vi "Pre Launch Init.vi"(11 "Popup ViewManager in":refnum<class "Popup ViewManager.lvclass">) -> (0 "error out":errorcluster, 3 "Popup ViewManager out":refnum<class "Popup ViewManager.lvclass">)   [LabVIEW 2019, in "Popup ViewManager.lvlib" / "Popup ViewManager.lvclass"]
doc: "(<B>Filename</B>: Actor Framework.lvlib:Actor.lvclass:Pre Launch Init.vi)\n\nDefines behavior that occurs after the Launch Nested Actor method is invoked but before the actor's Actor Core method begins running.\n\nBy default, this method does nothing. A descendant class may override it to define behavior."
uses:
  <vilib>/gpm_packages/@cs/popup-viewmanager/Source/Popup ViewManager/Popup ViewManager.lvclass
  C:/Program Files/National Instruments/LabVIEW 2019/vi.lib/ActorFramework/Actor/Actor.lvclass
  <vilib>/ActorFramework/Message Enqueuer/Message Priority.ctl
  <vilib>/ActorFramework/Actor/Actor.lvclass/Actor.ctl
  <vilib>/ActorFramework/Message Enqueuer/Message Enqueuer.lvclass/Message Enqueuer.ctl
  <vilib>/gpm_packages/@cs/popup-viewmanager/Source/Popup ViewManager/Popup ViewManager.lvclass/Popup ViewManager.ctl
  <vilib>/ActorFramework/Message Enqueuer/Init from Existing Queue.vi
  <vilib>/ActorFramework/Message Enqueuer/Enqueue.vi
  <vilib>/gpm_packages/@cs/popup-viewmanager/Source/Popup ViewManager Messages/Launch Nested Views Msg/Launch Nested Views Msg.lvclass
  C:/Program Files/National Instruments/LabVIEW 2019/vi.lib/ActorFramework/Message/Message.lvclass
  <vilib>/ActorFramework/Message Priority Queue/Priority Enqueue.vi
  <vilib>/gpm_packages/@cs/mva-dialogbox/source/IDialogBox/IDialogBox/IDialogBox.lvclass
  <vilib>/ActorFramework/Message Enqueuer/Message Enqueuer.lvclass
  <vilib>/ActorFramework/Actor/Actor.lvclass
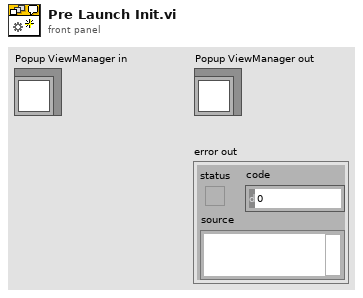
[diagram p1: front panel]
types:
  T1 = typedef "Actor Framework.lvlib/Message Enqueuer.lvclass/Message Priority.ctl" = enum16{"Low", "Normal", "High"}
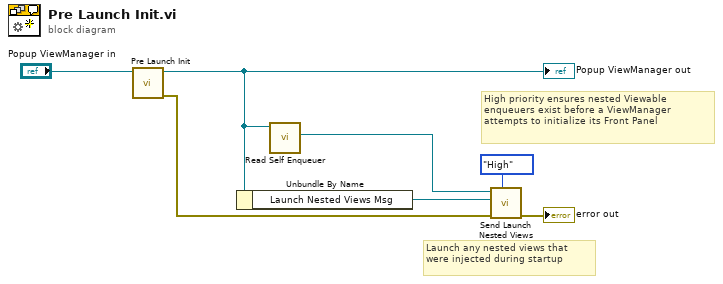
[diagram p0: block diagram]
diagram:
  # "Launch any nested views that\nwere injected during startup"
  # "High priority ensures nested Viewable\nenqueuers exist before a ViewManager\nattempts to initialize its Front Panel"
  n1 = call-parent "Pre Launch Init.vi"("IViewable in"="Popup ViewManager in") -> ("error out"=w4:errorcluster, "IViewable out"=w2:refnum<class "Popup ViewManager.lvclass">)  [unwired: 9 in]
  "Popup ViewManager out" <- w2
  n2 = Unbundle By Name(w2) -> ("Launch Nested Views Msg"=w1:refnum<class "Launch Nested Views Msg.lvclass">)
  n3 = call <vilib>:"Read Self Enqueuer.vi"("Actor"=w2) -> ("Self Enqueuer"=w6:refnum<class "Message Enqueuer.lvclass">)  [unwired: 10 in]
  n4 = call <vilib>:"Send Launch Nested Views.vi"("Message Priority (Normal)"=Message_Priority."High", "error in (no error)"=w4, "Launch Nested Views Msg"=w1, "Message Enqueuer"=w6) -> ("error out"=→"error out":errorcluster)  [unwired: 6 in, 1 out]
